vi "Wait with interrupt.vi"(9 "Tick count at loop start (ms)":u32, 11 "Loop iteration (ms)":u32=10000) -> ()   [LabVIEW 2017]
uses:
  Typedefs/Read Write Enum.ctl
panel:
  in  "millisecond multiple":u32=10
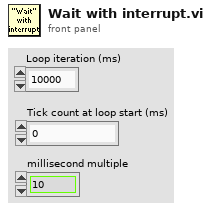
[diagram p1: front panel]
types:
  T1 = typedef "Read Write Enum.ctl" = enum16{"Read", "Write"}
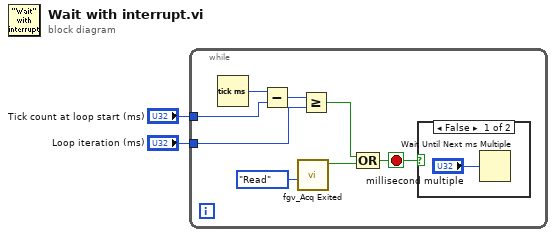
[diagram p0: block diagram]
diagram:
  n1 = while {
    tunnel: "Tick count at loop start (ms)" -> [w9]
    tunnel: "Loop iteration (ms)" -> [w7]
    stop <- w3 stop-if-true
    n2 = Tick Count (ms)() -> (millisecond timer value=w10:u32)
    n3 = Subtract(x=w10, y=w9) -> (x-y=w8:u32)
    n4 = call "fgv_Acq Exited.vi"("Function"=Read_Write_Enum."Read") -> ("Acquisition completed"=w4:bool)  [unwired: 9 in, 1 out]
    n5 = Greater Or Equal?(x=w8, y=w7) -> (x >= y?=w6:bool)
    n6 = Compound Arithmetic op=OR(w6, w4) -> (w3:bool)
    n7 = case shown="False" w3 {
      frame False {
        n8 = Wait Until Next ms Multiple(millisecond multiple="millisecond multiple") -> ()  [unwired: 1 out]
      }
      frame True {
      }
    }
  }
